vi "Adapt and Append Waveform.vi"(8 "Error":errorcluster, 9 "Raw Waveform":T1, 11 "WavBuf":refnum<class "WavBuf.lvclass">) -> (0 "Error Out":errorcluster, 3 "WavBuf Out":refnum<class "WavBuf.lvclass">, 5 "Left over Count":i32)   [LabVIEW 2025, in "WavBuf.lvclass"]
uses:
  WavBuf.lvclass
  Universal Controls/Waveform_Data.ctl
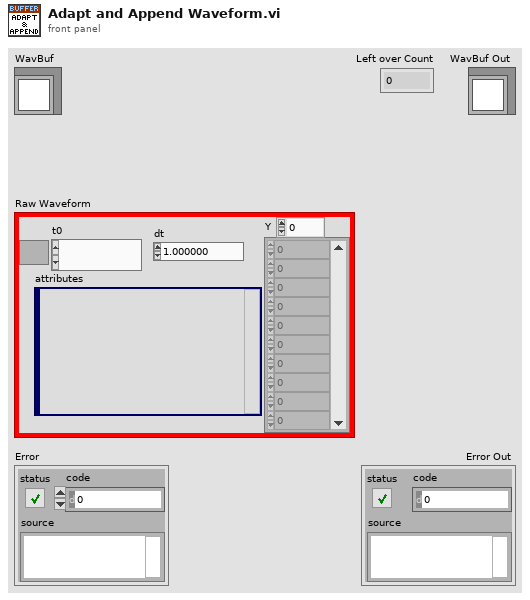
[diagram p1: front panel]
types:
  T1 = typedef "Waveform_Data.ctl" = waveform(dbl)
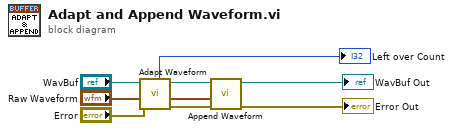
[diagram p0: block diagram]
diagram:
  n1 = call-dynamic "Adapt Waveform.vi"("Error"="Error", "Waveform"="Raw Waveform", "WavBuf"="WavBuf") -> ("Error Out"=w4:errorcluster, "Waveform Out"=w5:T1, "WavBuf Out"=w6:refnum<class "WavBuf.lvclass">, "Left over Count"=→"Left over Count":i32)  [unwired: 5 in]
  n2 = call "Append Waveform.vi"("Error"=w4, "Waveform To Append"=w5, "WavBuf"=w6) -> ("Error Out"=→"Error Out":errorcluster, "WavBuf Out"=→"WavBuf Out":refnum<class "WavBuf.lvclass">)  [unwired: 6 in, 1 out]
